vi "Initiate Updates.vi"(8 "error in (no error)":errorcluster, 11 "Popup ViewManager In":refnum<class "Popup ViewManager.lvclass">) -> (0 "error out":errorcluster, 3 "Popup ViewManager Out":refnum<class "Popup ViewManager.lvclass">)   [LabVIEW 2019, in "Popup ViewManager.lvlib" / "Popup ViewManager.lvclass"]
doc: "<License>\nCopyright © 2017 Composed Systems, LLC | All rights reserved\nwww.composed.io\n\nAuthor: Ethan Stern <ethan.stern@composed.io>\n\nThis software is provided \"AS IS\" WITHOUT WARRANTIES, either express or implied, AND IS FOR EDUCATIONAL PURPOSES ONLY.\n</License>"
uses:
  <vilib>/gpm_packages/@cs/popup-viewmanager/Source/Popup ViewManager/Popup ViewManager.lvclass
  C:/Program Files/National Instruments/LabVIEW 2019/vi.lib/gpm_packages/@cs/mva-viewable/Source/IViewable/IViewable/IViewable.lvclass
  <vilib>/gpm_packages/@cs/mva-viewable/Source/IViewable/IViewable/IViewable.lvclass/IViewable.ctl
  <vilib>/gpm_packages/@cs/popup-viewmanager/Source/Popup ViewManager/Popup ViewManager.lvclass/Popup ViewManager.ctl
  <vilib>/gpm_packages/@cs/mva-viewable/Source/IViewable/IViewable/IViewable.lvclass
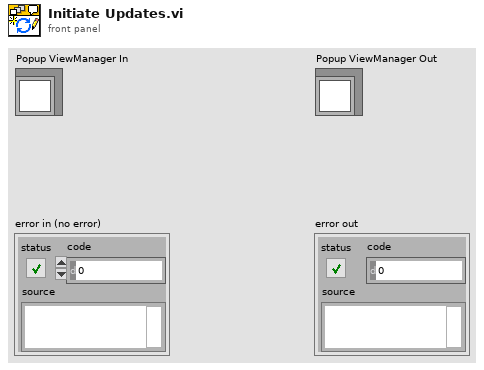
[diagram p1: front panel]
types:
  T1 = enum32{"Invalid", "Default", "Floating", "Floating/Auto-Hide", "Modal"}
  T2 = enum32{"Invalid", "Standard", "Closed", "Hidden", "Minimized", "Maximized"}
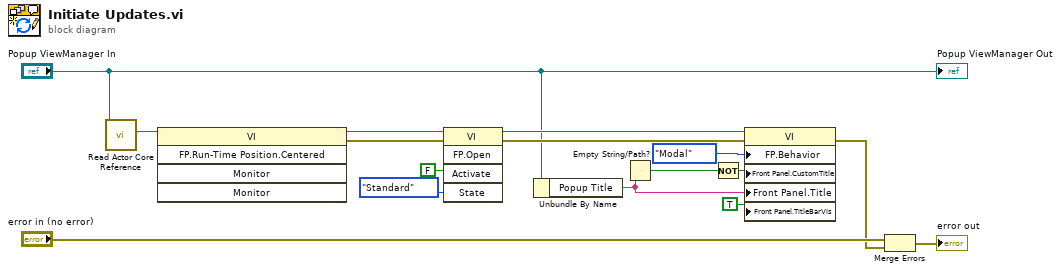
[diagram p0: block diagram]
diagram:
  n1 = call <vilib>:"Read Actor Core Reference.vi"("IViewable In"="Popup ViewManager In") -> ("Actor Core Refnum"=w15:refnum<vi>)  [unwired: 9 in, 1 out]
  n2 = invoke class="VI" method="FP.Run-Time Position.Centered"(reference=w15) -> (reference out=w11:refnum<vi>, error out=w10:errorcluster)  [unwired: 4 in, 3 out]
  n3 = invoke class="VI" method="FP.Open"(reference=w11, error in=w10, "Activate"=FALSE ("Activate?"), "State"=T2."Standard") -> (reference out=w8:refnum<vi>, error out=w7:errorcluster)  [unwired: 1 in, 3 out]
  n4 = Unbundle By Name("Popup ViewManager In") -> ("Popup Title"=w3:string)
  n5 = Empty String/Path?(string/path=w3) -> (empty?=w2:bool)
  n6 = Not(x=w2) -> (.not. x?=w1:bool)
  n7 = property class="VI"(reference=w8, error in=w7, "FP.Behavior"=T1."Modal" ("Front Panel Window:Behavior"), "Front Panel.CustomTitle"=w1, "Front Panel.Title"=w3, "Front Panel.TitleBarVis"=TRUE ("Front Panel Window:Title Bar Visible")) -> (error out=w6:errorcluster)  [unwired: 1 out]
  n8 = Merge Errors("error in (no error)", w6) -> (→"error out":errorcluster)
  "Popup ViewManager Out" <- "Popup ViewManager In"
